vi "process-init.vi"(0 "Process In":refnum<vi>, 5 "Parameter":refnum<vi>, 7 "Time":dbl=100.0, 11 "Error In":errorcluster) -> (4 "Process Out":refnum<vi>, 6 "Parameter out":refnum<vi>, 15 "Error Out":errorcluster)   [LabVIEW 2016]
uses:
  controls/Parameters.ctl
  controls/Lambda.ctl
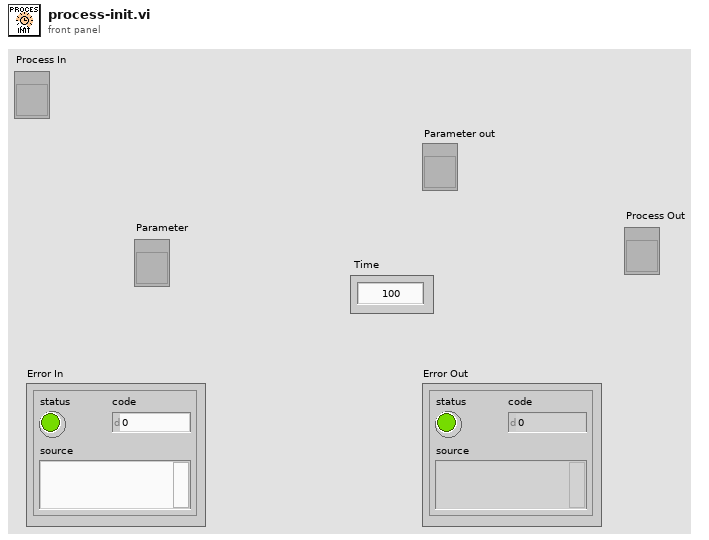
[diagram p1: front panel]
types:
  T1 = typedef "Parameters.ctl" = cluster{"Lambda":T2, "Power":dbl, "Frequency":dbl, "Stabilizing":dbl, "Samples":dbl, "File":path}
  T2 = typedef "Lambda.ctl" = cluster{"Init":dbl, "Final":dbl, "dx":dbl}
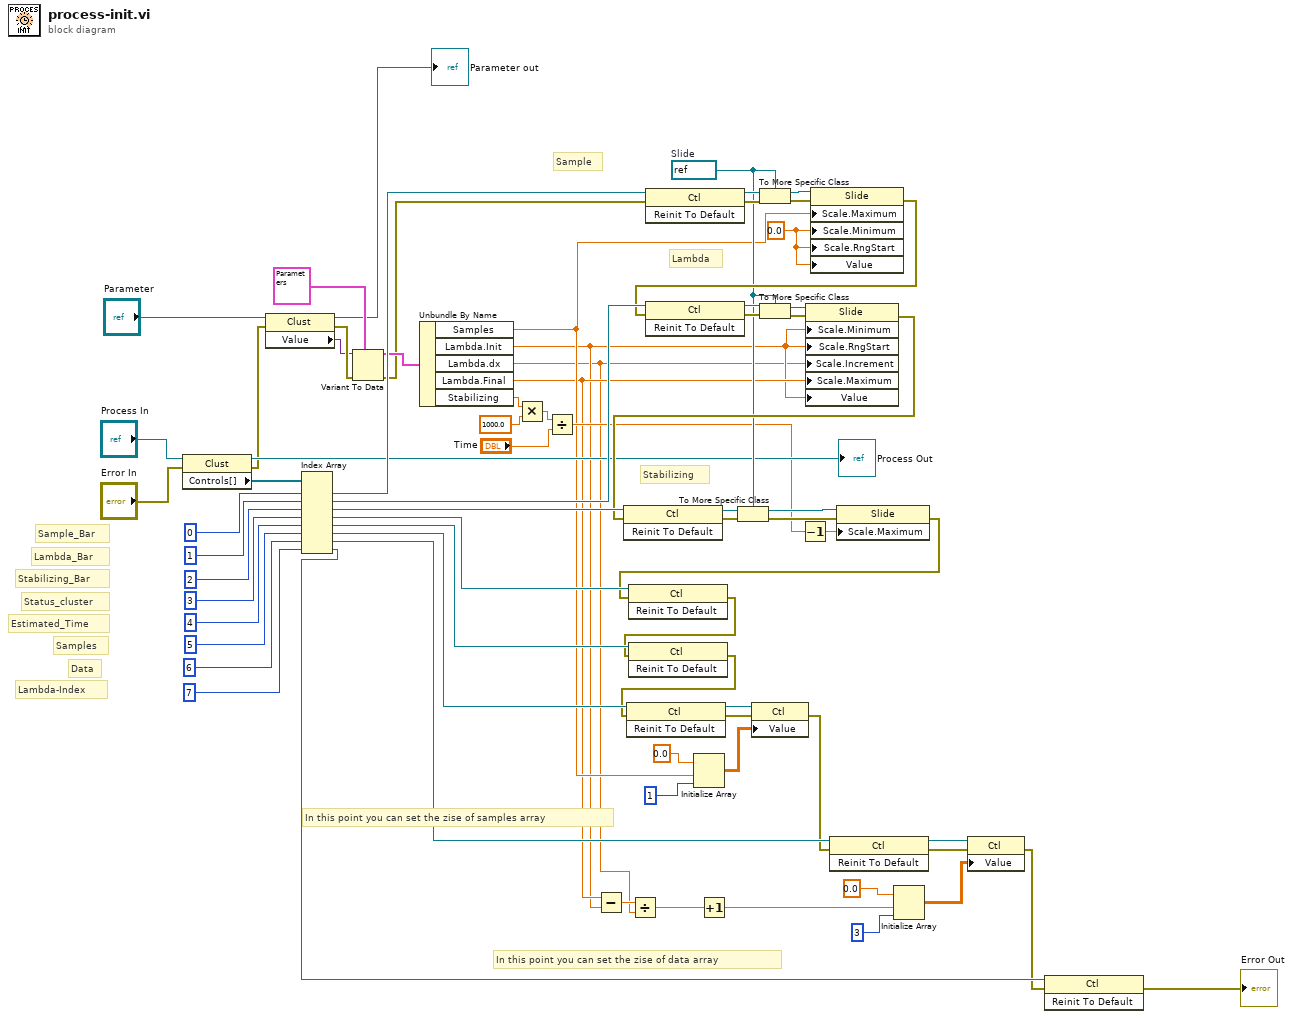
[diagram p0: block diagram]
diagram:
  w40 = 0.0 ("Scale.Range:Minimum")
  w45 = refnum<vi> refnum  # Slide
  # "Lambda-Index"
  # "In this point you can set the zise of data array"
  # "Data"
  # "In this point you can set the zise of samples array"
  # "Samples"
  # "Stabilizing"
  # "Lambda"
  # "Sample"
  # "Estimated_Time"
  # "Status_cluster"
  # "Stabilizing_Bar"
  # "Lambda_Bar"
  # "Sample_Bar"
  n1 = property class="Clust"(reference="Process In", error in="Error In") -> (reference out=→"Process Out":refnum<vi>, error out=w26:errorcluster, "Controls[]"=w71:refnum<vi>[])
  n2 = property class="Clust"(reference="Parameter", error in=w26) -> (reference out=→"Parameter out":refnum<vi>, error out=w24:errorcluster, "Value"=w23:variant)
  n3 = Index Array(array=w71, index #1=0, index #2=1, index #3=2, index #4=3, index #5=4, index #6=5, index #7=6 ("index"), index #8=7) -> (element #1=w65:refnum<vi>, element #2=w64:refnum<vi>, element #3=w63:refnum<vi>, element #4=w62:refnum<vi>, element #5=w61:refnum<vi>, element #6=w38:refnum<vi>, element #7=w18:refnum<vi>, element #8=w6:refnum<vi>)
  n4 = Variant To Data(error in=w24, type=T1 {"Lambda"={"Init"=0.0, "Final"=0.0, "dx"=0.0}, "Power"=0.0, "Frequency"=0.0, "Stabilizing"=0.0, "Samples"=0.0, "File"=path ""} ("Parameters"), Variant=w23) -> (data=w21:T1, error out=w20:errorcluster)
  n5 = Unbundle By Name(w21) -> ("Samples"=w33:dbl, "Lambda.Init"=w12:dbl, "Lambda.dx"=w10:dbl, "Lambda.Final"=w13:dbl, "Stabilizing"=w31:dbl)
  n6 = Multiply(x=w31, y=1000.0) -> (x*y=w29:dbl)
  n7 = Divide(x=w29, y="Time") -> (x/y=w41:dbl)
  n8 = Subtract(x=w13, y=w12) -> (x-y=w11:dbl)
  n9 = Divide(x=w11, y=w10) -> (x/y=w3:dbl)
  n10 = invoke class="Ctl" method="Reinit To Default"(reference=w65, error in=w20) -> (reference out=w60:refnum<vi>, error out=w59:errorcluster)  [unwired: 1 in, 1 out]
  n11 = Initialize Array(0.0, w33, 1 ("dimension size")) -> (w32:dbl[][])
  n12 = Increment(x=w3) -> (x+1=w2:dbl)
  n13 = To More Specific Class(target class=w45, reference=w60, error in=w59) -> (specific class reference=w58:refnum<vi>, error out=w57:errorcluster)
  n14 = Decrement(x=w41) -> (x-1=w42:dbl)
  n15 = property class="Slide"(reference=w58, error in=w57, "Scale.Maximum"=w33, "Scale.Minimum"=w40, "Scale.RngStart"=w40, "Value"=w40) -> (error out=w52:errorcluster)  [unwired: 1 out]
  n16 = invoke class="Ctl" method="Reinit To Default"(reference=w64, error in=w52) -> (reference out=w56:refnum<vi>, error out=w55:errorcluster)  [unwired: 1 in, 1 out]
  n17 = To More Specific Class(target class=w45, reference=w56, error in=w55) -> (specific class reference=w54:refnum<vi>, error out=w53:errorcluster)
  n18 = property class="Slide"(reference=w54, error in=w53, "Scale.Minimum"=w12, "Scale.RngStart"=w12, "Scale.Increment"=w10, "Scale.Maximum"=w13, "Value"=w12) -> (error out=w47:errorcluster)  [unwired: 1 out]
  n19 = invoke class="Ctl" method="Reinit To Default"(reference=w63, error in=w47) -> (reference out=w51:refnum<vi>, error out=w50:errorcluster)  [unwired: 1 in, 1 out]
  n20 = To More Specific Class(target class=w45, reference=w51, error in=w50) -> (specific class reference=w49:refnum<vi>, error out=w48:errorcluster)
  n21 = property class="Slide"(reference=w49, error in=w48, "Scale.Maximum"=w42) -> (error out=w46:errorcluster)  [unwired: 1 out]
  n22 = invoke class="Ctl" method="Reinit To Default"(reference=w62, error in=w46) -> (error out=w44:errorcluster)  [unwired: 1 in, 2 out]
  n23 = invoke class="Ctl" method="Reinit To Default"(reference=w61, error in=w44) -> (error out=w37:errorcluster)  [unwired: 1 in, 2 out]
  n24 = invoke class="Ctl" method="Reinit To Default"(reference=w38, error in=w37) -> (reference out=w36:refnum<vi>, error out=w35:errorcluster)  [unwired: 1 in, 1 out]
  n25 = property class="Ctl"(reference=w36, error in=w35, "Value"=w32) -> (error out=w17:errorcluster)  [unwired: 1 out]
  n26 = invoke class="Ctl" method="Reinit To Default"(reference=w18, error in=w17) -> (reference out=w16:refnum<vi>, error out=w15:errorcluster)  [unwired: 1 in, 1 out]
  n27 = Initialize Array(0.0 ("element"), w2, 3 ("dimension size")) -> (w8:dbl[][])
  n28 = property class="Ctl"(reference=w16, error in=w15, "Value"=w8) -> (error out=w5:errorcluster)  [unwired: 1 out]
  n29 = invoke class="Ctl" method="Reinit To Default"(reference=w6, error in=w5) -> (error out=→"Error Out":errorcluster)  [unwired: 1 in, 2 out]
